vi "FGV_states_2D.vi"(8 "error in":errorcluster, 9 "device, col":T2, 10 "status, row":T1, 11 "action":T3=enum."read") -> (0 "error out":errorcluster, 1 "bit_state":bool, 2 "states of requested device":bool[](array[boolean]), 3 "devices with requested status":bool[](array[boolean]), 4 "2Dstate":bool[][](array[boolean]), 5 "Devices []":string[](array[string])=["Huber", "Azura", "Foxy", "DMM", "PS1", "PS2", "PS3", "PS4", "K1", "K2", "K3"], 7 "States":string[](array[string])=["Huber", "Azura", "Foxy", "DMM", "PS1", "PS2", "PS3", "PS4", "K1", "K2", "K3"])   [LabVIEW 2018]
uses:
  controls/2D_action.ctl
  controls/2D_devices.ctl
  controls/2D_status.ctl
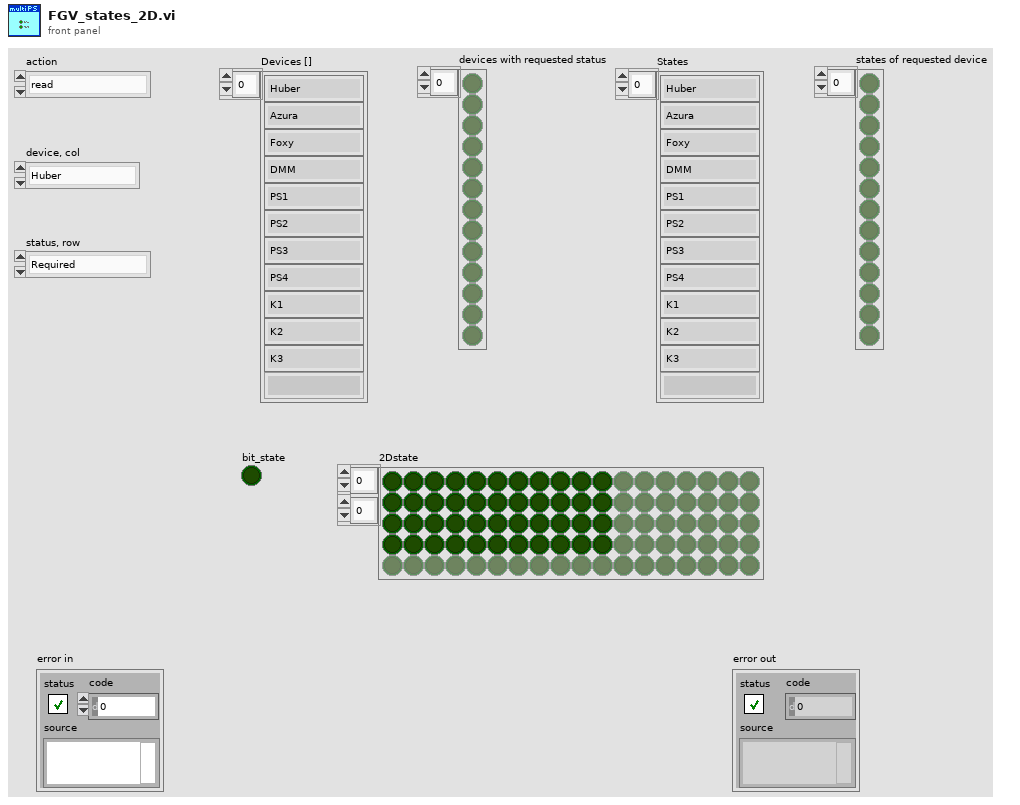
[diagram p1: front panel]
types:
  T1 = typedef "2D_status.ctl" = enum16{"Required", "Initialized", "In Use", "In Error"}
  T2 = typedef "2D_devices.ctl" = enum16{"Huber", "Azura", "Foxy", "DMM", "PS1", "PS2", "PS3", "PS4", "K1", "K2", "K3"}
  T3 = typedef "2D_action.ctl" = enum16{"init", "set bit", "clear bit", "read"}
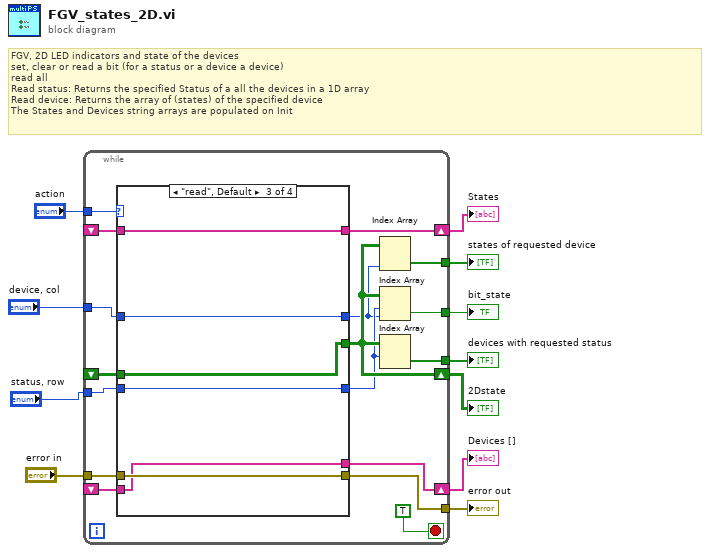
[diagram p0: block diagram]
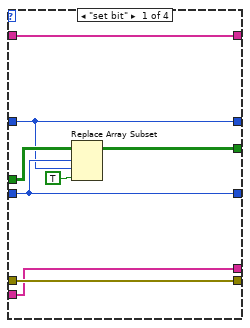
[diagram p2: hidden frame]
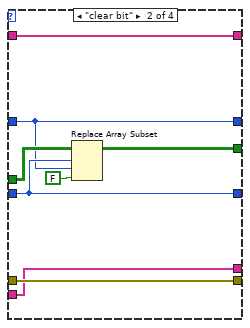
[diagram p3: hidden frame]
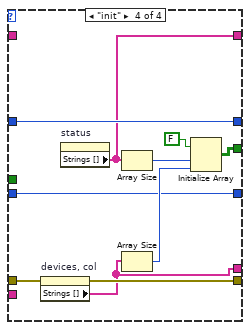
[diagram p4: hidden frame]
diagram:
  # "FGV, 2D LED indicators and state of the devices\nset, clear or read a bit (for a status or a device a device)\nread all\nRead status: Returns the specified Status of a all the devices in a 1D array\nRead device: Returns the array of (states) of the specified device\nThe States and Devices string arrays are populated on Init"
  n1 = while {
    tunnel: "action" -> [w28]
    tunnel: "device, col" -> [w17]
    tunnel: "status, row" -> [w19]
    shift-right: [w21] -> w6
    shift-left: _ -> [w25]
    tunnel: [w23] -> w5
    tunnel: [w22] -> w4
    tunnel: [w20] -> w3
    shift-right: [w14] -> w1
    shift-left: _ -> [w13]
    shift-right: [w15] -> w2
    shift-left: _ -> [w12]
    tunnel: "error in" -> [w26]
    tunnel: [w24] -> w8
    stop <- TRUE stop-if-true
    n2 = case shown="\"read\", Default" w28 {
      tunnel: w26 -> [w36 w44 w50 w59]
      tunnel: [w36 w44 w50 w60] -> w24
      tunnel: [w33 w41 w49 w55] -> w21
      tunnel: w25 -> [w35 w43 w49 _]
      tunnel: w19 -> [w32 w40 w48 w54]
      tunnel: w17 -> [w31 w39 w47 w53]
      tunnel: [w32 w40 w48 w54] -> w18
      tunnel: [w31 w39 w47 w53] -> w16
      tunnel: [w29 w37 w45 w52] -> w15
      tunnel: [w30 w38 w46 w51] -> w14
      tunnel: w13 -> [w30 w38 w46 _]
      tunnel: w12 -> [w29 w37 w45 _]
      frame "set bit" {
        n3 = Replace Array Subset(array=w35, new element=TRUE ("new element/subarray"), index (row)=w32, index (col)=w31) -> (w33:bool[][])
      }
      frame "clear bit" {
        n4 = Replace Array Subset(array=w43, new element=FALSE ("new element/subarray"), index (row)=w40, index (col)=w39) -> (w41:bool[][])
      }
      frame "read", Default {
      }
      frame "init" {
        n5 = property on="devices, col" class="Enum (strict)"(error in=w59) -> (error out=w60:errorcluster, "Strings []"=w52:string[])  [unwired: 1 in, 1 out]
        n6 = property on="status" class="Enum (strict)"() -> ("Strings []"=w51:string[])  [unwired: 2 in, 2 out]
        n7 = Array Size(array=w51) -> (size(s)=w56:i32)
        n8 = Array Size(array=w52) -> (size(s)=w57:i32)
        n9 = Initialize Array(FALSE, w56, w57) -> (w55:bool[][])
      }
    }
    n10 = Index Array(array=w21, index (col)=w16) -> (element=w23:bool[])  [unwired: 1 in]
    n11 = Index Array(array=w21, index (row)=w18, index (col)=w16) -> (element=w22:bool)
    n12 = Index Array(array=w21, index (row)=w18) -> (element=w20:bool[])  [unwired: 1 in]
  }
  "error out" <- w8
  "2Dstate" <- w6
  "states of requested device" <- w5
  "bit_state" <- w4
  "devices with requested status" <- w3
  "Devices []" <- w2
  "States" <- w1
